vi "L1_BaselineTest_File_Create.vi"(1 "input cluster":T1, 2 "Serial Number":string="testFile") -> (0 "appended path":path)   [LabVIEW 2012]
uses:
  <vilib>/Utility/NIReport.llb/NI_report.lvclass
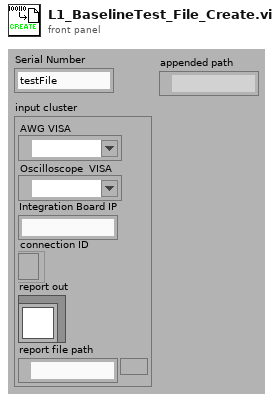
[diagram p1: front panel]
types:
  T1 = cluster{"AWG VISA":refnum<visa-resource-name>, "Oscilloscope  VISA ":refnum<visa-resource-name>, "Integration Board IP":string, "connection ID":refnum<k5>, "report out":refnum<class "NI_report.lvclass">, "report file path":path}
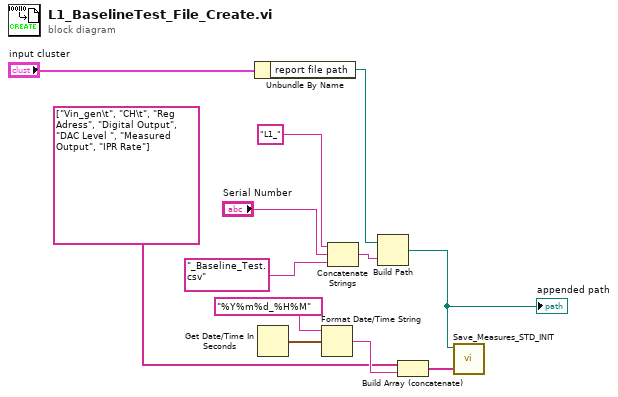
[diagram p0: block diagram]
diagram:
  n1 = Unbundle By Name("input cluster") -> ("report file path"=w6:path)
  n2 = Get Date/Time In Seconds() -> (seconds since 1Jan1904=w11:timestamp)
  n3 = Format Date/Time String(time format string (%c)="%Y%m%d_%H%M", seconds (now)=w11) -> (date/time string=w9:string)  [unwired: 1 in]
  n4 = Concatenate Strings("L1_" ("format string"), "Serial Number", "_Baseline_Test.csv" ("format string")) -> (w7:string)
  n5 = Build Path(base path=w6, name or relative path=w7) -> (appended path=w4:path)
  "appended path" <- w4
  n6 = Build Array (concatenate)(string[] ["Vin_gen\t", "CH\t", "Reg Adress", "Digital Output", "DAC Level ", "Measured Output", "IPR Rate"] ("appended array"), w9) -> (w12:string[])
  n7 = call "Save_Measures_STD_INIT.vi"("appended array"=w12, "file path (dialog if empty)"=w4) -> ()  [unwired: 10 in]
